vi "NML SCM IPS make persistent.vi"(0 "VISA session":refnum<visa-resource-name>="GPIB0::22::INSTR", 1 "Input Cluster":T1 {"MaxLambdaCurrent [A]" format="%.2f"; "LambdaRates [A/min]" format="%.5e"; "MaxNormalCurrent [A]" format="%.2f"; "StabilitySetting [%]" format="%.2f"; "FieldCurrentRatio [T/A]" format="%.2f"; "SwitchWaitTime [s]" format="%.2f"; "SwitchHtrCurrent [mA]" format="%.2f"; "TrainRates [A/min]" format="%.5e"; "NormalRates [A/min]" format="%.5e"; "Breakpts [A]" format="%.5e"}) -> (2 "dup VISA session":refnum<visa-resource-name>, 3 "Persistence Field":dbl format="%.2f", 4 "String":string, 5 "Persistence Out":bool=TRUE)   [LabVIEW 2019]
uses:
  Instance           6 35Saved   NML SCM IPS make persistant .vi
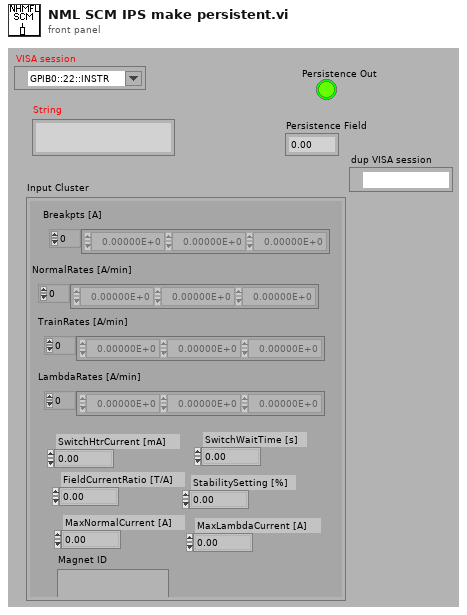
[diagram p1: front panel]
types:
  T1 = cluster{"Breakpts [A]":dbl[], "NormalRates [A/min]":dbl[], "TrainRates [A/min]":dbl[], "SwitchHtrCurrent [mA]":dbl, "SwitchWaitTime [s]":dbl, "FieldCurrentRatio [T/A]":dbl, "StabilitySetting [%]":dbl, "MaxNormalCurrent [A]":dbl, "Magnet ID":string, "LambdaRates [A/min]":dbl[], "MaxLambdaCurrent [A]":dbl}
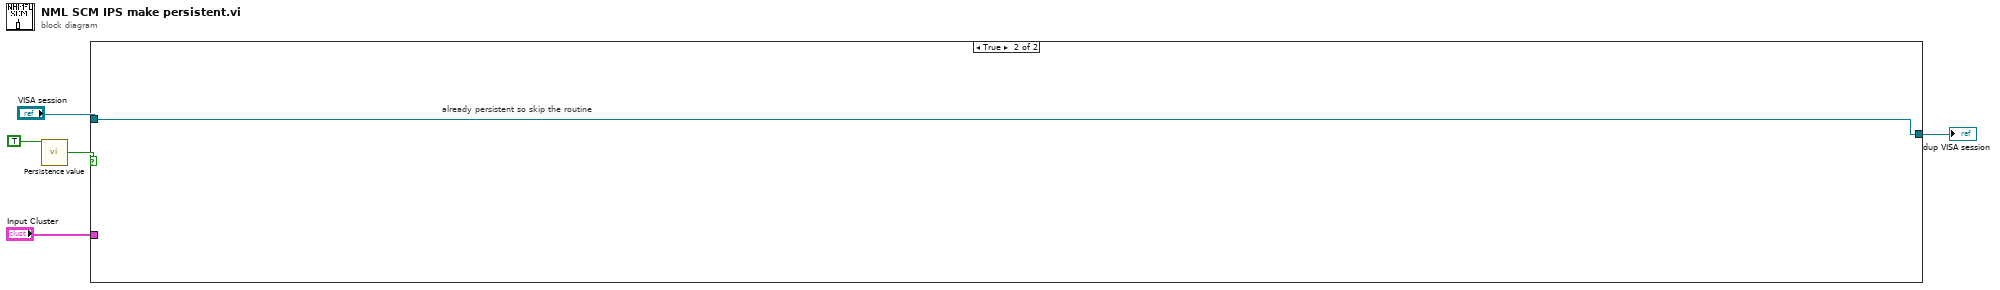
[diagram p0: block diagram]
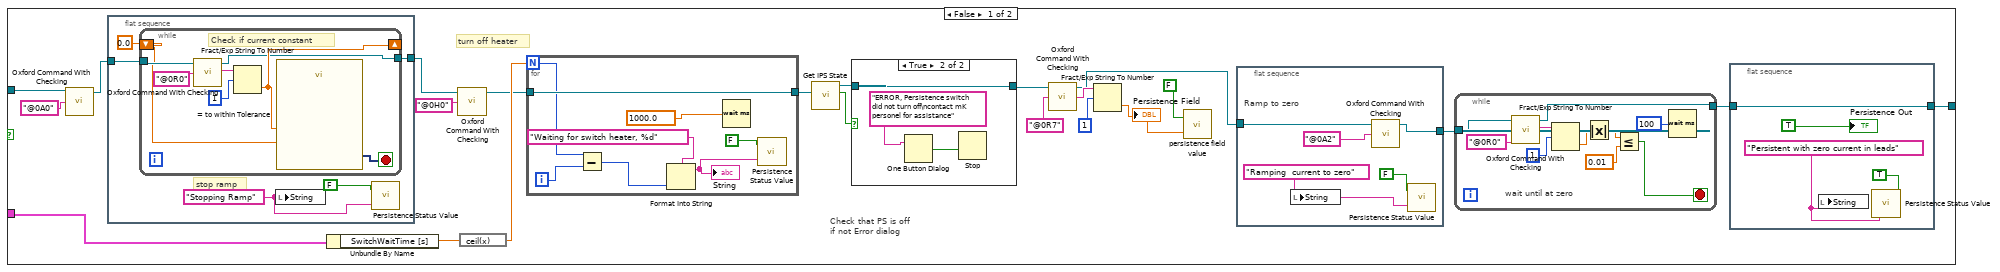
[diagram p2: hidden frame]
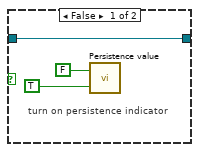
[diagram p3: hidden frame]
diagram:
  n1 = call "Persistence value.vi"("Read/Write this vi"=TRUE ("Read/Write")) -> ("Persistence Out"=w4:bool)  [unwired: 1 in]
  n2 = case shown="True" w4 {
    tunnel: "VISA session" -> [w10 w74]
    tunnel: "Input Cluster" -> [w24 _]
    tunnel: [w6 w74] -> w1
    frame False {
      # "turn off heater"
      # "Check that PS is off \nif not Error dialog"
      n3 = call "Oxford Command With Checking.vi"("Command"="@0A0", "VISA session"=w10) -> ("dup VISA session"=w9:refnum<visa-resource-name>)  [unwired: 1 in, 2 out]
      n4 = flat-sequence {
        tunnel: w9 -> [w30]
        tunnel: [w28] -> w7
        frame #0 {
          w31 = "Stopping Ramp"
          # "stop ramp"
          n5 = while {
            tunnel: w30 -> [w38]
            shift-right: [w34] -> _
            shift-left: 0.0 -> [w36]
            tunnel: [w33] -> w28
            stop <- w35 stop-if-true
            # "Check if current constant"
            n6 = call "Oxford Command With Checking.vi"("Command"="@0R0", "VISA session"=w38) -> ("String Read"=w40:string, "dup VISA session"=w33:refnum<visa-resource-name>)  [unwired: 1 in, 1 out]
            n7 = Fract/Exp String To Number(string=w40, offset=1) -> (number=w34:dbl)  [unwired: 2 in, 1 out]
            n8 = call "= to within Tolerance"("Constant Value to Compare Against"=w36, "Operand 1"=w34) -> ("Result"=w35:dynamicdata)  [unwired: 8 in, 1 out]
          }
          n9 = local write "String"(w31) -> ()
          n10 = call "Persistence Status Value.vi"("Persistence Status In"=w31, "Read/Write this vi"=FALSE) -> ()  [unwired: 1 out]
        }
      }
      n11 = Unbundle By Name(w24) -> ("SwitchWaitTime [s]"=w23:dbl)
      n12 = call "Oxford Command With Checking.vi"("Command"="@0H0", "VISA session"=w7) -> ("dup VISA session"=w21:refnum<visa-resource-name>)  [unwired: 1 in, 2 out]
      n13 = expression code="ceil(x)"(w23) -> (w22:dbl)
      n14 = for {
        N: w22 -> [w51]
        tunnel: w21 -> [w54]
        tunnel: [w54] -> w20
        i -> [w52]
        n15 = Subtract(x=w51, y=w52) -> (x-y=w50:i32)
        n16 = Format Into String(format string="Waiting for switch heater, %d", w50) -> (resulting string=w56:string)  [unwired: 2 in, 1 out]
        "String" <- w56
        n17 = Wait (ms)(milliseconds to wait=1000.0 ("y")) -> ()  [unwired: 1 out]
        n18 = call "Persistence Status Value.vi"("Persistence Status In"=w56, "Read/Write this vi"=FALSE) -> ()  [unwired: 1 out]
      }
      n19 = call "Get IPS State.vi"("VISA session"=w20) -> ("dup VISA session"=w18:refnum<visa-resource-name>, "Switch Heater"=w19:bool)  [unwired: 1 in, 3 out]
      n20 = case shown="True" w19 {
        tunnel: w18 -> [w70 w71]
        tunnel: [w70 w71] -> w16
        frame False {
          # "turn on persistence indicator"
          n21 = call "Persistence value.vi"("Persistence In"=TRUE, "Read/Write this vi"=FALSE) -> ()  [unwired: 1 out]
        }
        frame True {
          n22 = One Button Dialog(message="ERROR, Persistence switch did not turn off\ncontact mK personel for assistance") -> (true=w72:bool)  [unwired: 1 in]
          n23 = Stop(stop? (T)=w72) -> ()
        }
      }
      n24 = call "Oxford Command With Checking.vi"("Command"="@0R7" ("Command String"), "VISA session"=w16) -> ("String Read"=w15:string, "dup VISA session"=w8:refnum<visa-resource-name>)  [unwired: 1 in, 1 out]
      n25 = Fract/Exp String To Number(string=w15, offset=1) -> (number=w13:dbl)  [unwired: 2 in, 1 out]
      "Persistence Field" <- w13
      n26 = call "persistence field value.vi"("Persistent Field In"=w13, "Read/Write this vi"=FALSE) -> ()  [unwired: 1 out]
      n27 = flat-sequence {
        tunnel: w8 -> [w47]
        tunnel: [w45] -> w12
        frame #0 {
          w49 = "Ramping  current to zero" ("String")
          # "Ramp to zero"
          n28 = local write "String"(w49) -> ()
          n29 = call "Oxford Command With Checking.vi"("Command"="@0A2" ("String to Write"), "VISA session"=w47) -> ("dup VISA session"=w45:refnum<visa-resource-name>)  [unwired: 1 in, 2 out]
          n30 = call "Persistence Status Value.vi"("Persistence Status In"=w49, "Read/Write this vi"=FALSE) -> ()  [unwired: 1 out]
        }
      }
      n31 = while {
        tunnel: w12 -> [w65]
        tunnel: [w58] -> w11
        stop <- w59 stop-if-true
        # "wait until at zero"
        n32 = call "Oxford Command With Checking.vi"("Command"="@0R0", "VISA session"=w65) -> ("String Read"=w64:string, "dup VISA session"=w58:refnum<visa-resource-name>)  [unwired: 1 in, 1 out]
        n33 = Fract/Exp String To Number(string=w64, offset=1) -> (number=w61:dbl)  [unwired: 2 in, 1 out]
        n34 = Absolute Value(x=w61) -> (abs(x)=w62:dbl)
        n35 = Less Or Equal?(x=w62, y=0.01) -> (x <= y?=w59:bool)
        n36 = Wait (ms)(milliseconds to wait=u32 100) -> ()  [unwired: 1 out]
      }
      n37 = flat-sequence {
        tunnel: w11 -> [w41]
        tunnel: [w41] -> w6
        frame #0 {
          w43 = "Persistent with zero current in leads" ("String")
          n38 = local write "String"(w43) -> ()
          n39 = call "Persistence Status Value.vi"("Persistence Status In"=w43, "Read/Write this vi"=TRUE) -> ()  [unwired: 1 out]
          "Persistence Out" <- TRUE
        }
      }
    }
    frame True {
      # "already persistent so skip the routine"
    }
  }
  "dup VISA session" <- w1
